vi "ATS_AbortCapture.vi"(11 "DeviceIn":i32) -> (0 "Return Code":u32, 3 "DeviceOut":i32, 5 "#Device":i32)   [LabVIEW 2015]
doc: "_____AlazarTech, Scope_____\n\nForce the device to abort the capture."
uses:
  ATS_ctl/ATS_Global_Ctrl.ctl
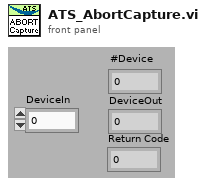
[diagram p1: front panel]
types:
  T1 = typedef "ATS_Global_Ctrl.ctl" = enum16{"Init_Device", "Clear_ALL", "Set", "Get"}
  T2 = typedef "Device_Info.ctl" = cluster{"Handle":u32, "Board":string, "CPLD":string, "MemorySize":u32, "SampleSize":u8, "ID":i32, "High_Memory":bool, "Chan/Board":u8}
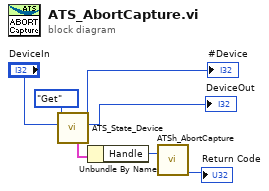
[diagram p0: block diagram]
diagram:
  n1 = call "ATS_State_Device.vi"("DeviceIn"="DeviceIn", "ATS_GBL_Ctrl"=ATS_Global_Ctrl."Get") -> ("DeviceOut"=→"DeviceOut":i32, "#Device"=→"#Device":i32, "DevInfo_Out"=w4:T2)  [unwired: 4 in, 3 out]
  n2 = Unbundle By Name(w4) -> ("Handle"=w1:u32)
  n3 = call "ATSh_AbortCapture.vi"("Handle"=w1) -> ("Return Code"=→"Return Code":u32)  [unwired: 9 in, 1 out]
